vi "Override Error.vi"(10 "Error":errorcluster, 11 "Dev Panel in":refnum<class "Dev Panel.lvclass">) -> (3 "Dev Panel out":refnum<class "Dev Panel.lvclass">)   [LabVIEW 2021, in "Dev Panel.lvclass"]
uses:
  Dev Panel.lvclass
  Dev Panel.lvclass/Dev Panel.ctl
  Actor/Event Actor/Event Actor.lvclass
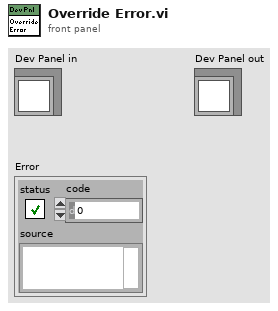
[diagram p1: front panel]
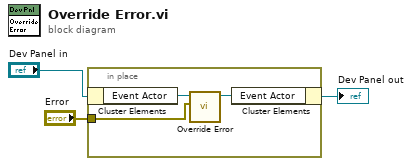
[diagram p0: block diagram]
diagram:
  n1 = in-place {
    in-place-border: "Error" -> [w4]
    n2 = in-place-cluster #1("Dev Panel in") -> ("Event Actor"=w6:refnum<class "Event Actor.lvclass">)
    n3 = call-dynamic "Override Error.vi"("Error"=w4, "Override Error in"=w6) -> ("Override Error out"=w5:refnum<class "Event Actor.lvclass">)  [unwired: 9 in]
    n4 = in-place-cluster #1("Event Actor"=w5) -> (→"Dev Panel out":refnum<class "Dev Panel.lvclass">)
  }
